vi "Database Configuration Import and Export and Refesh.vi"(8 "error in (no error)":errorcluster, 10 "Database Configuration":T1(ring), 11 "Settings in":refnum<class "Settings.lvclass">) -> (0 "error out":errorcluster, 3 "Settings out":refnum<class "Settings.lvclass">)   [LabVIEW 2023, in "GUI.lvlib" / "Settings.lvlib" / "Settings.lvclass"]
uses:
  Settings.lvclass
  HardwareAbstractionLayer_LVOOP/Database/SQL Public VI/Control/DB Options.ctl
  Settings.lvclass/Settings.ctl
  <vilib>/Utility/file.llb/Read Delimited Spreadsheet (string).vi
  <vilib>/Utility/file.llb/Write Delimited Spreadsheet (string).vi
  HardwareAbstractionLayer_LVOOP/Database/Database.lvclass
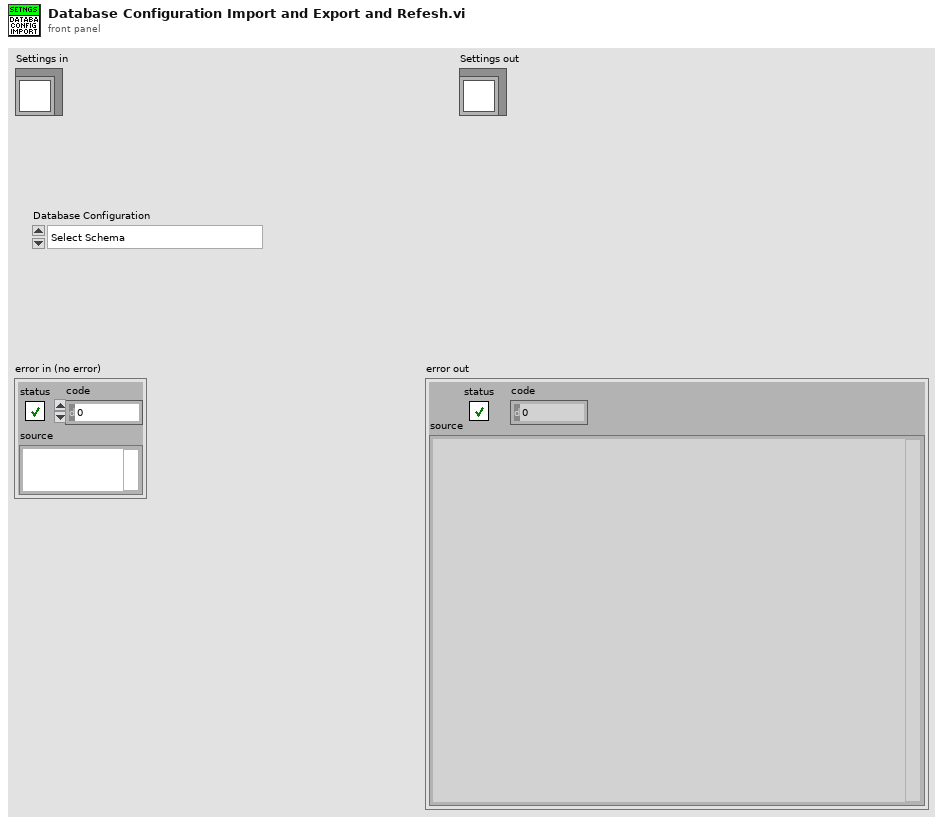
[diagram p1: front panel]
types:
  T1 = enum16{"Select Schema", "Select Table", "Import Table", "Export Table", "Refresh"}
  T2 = typedef "HardwareAbstractionLayer_LVOOP.lvlib/Database.lvclass/DB Options.ctl" = enum16{"Init", "Select Data", "Insert Data", "Update Data", "Delete Data", "Execute Query", "Create Schema", "Create Table", "List Tables", "List Columns", "Close"}
  T3 = cluster{"table":string, "columns":string[], "Data":string[][], "Schema Name":string}
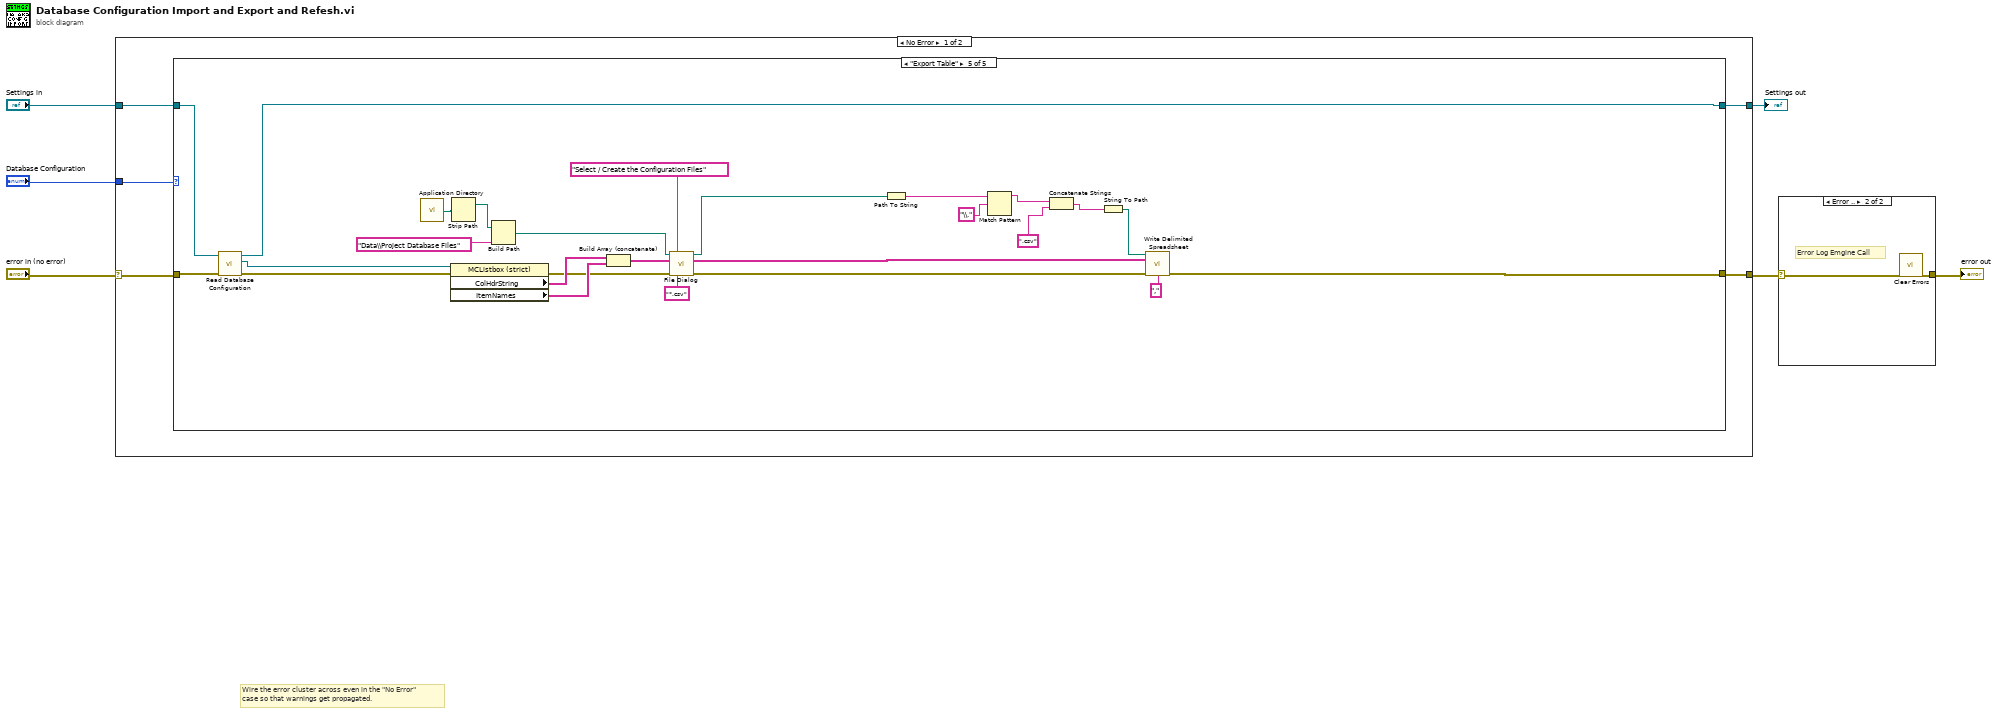
[diagram p0: block diagram]
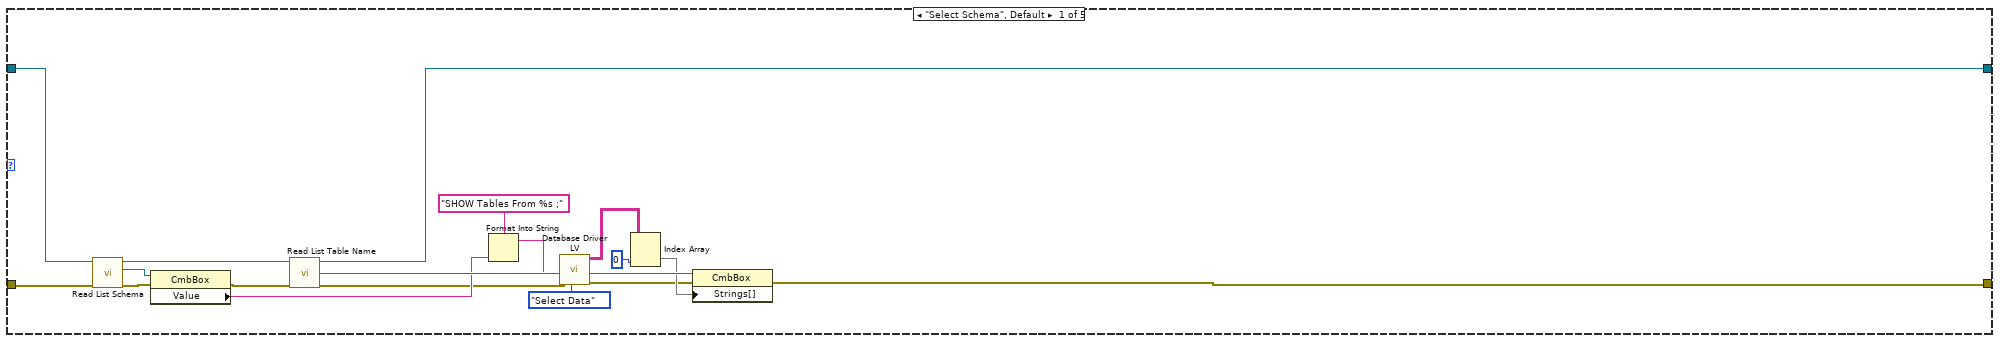
[diagram p3: hidden frame]
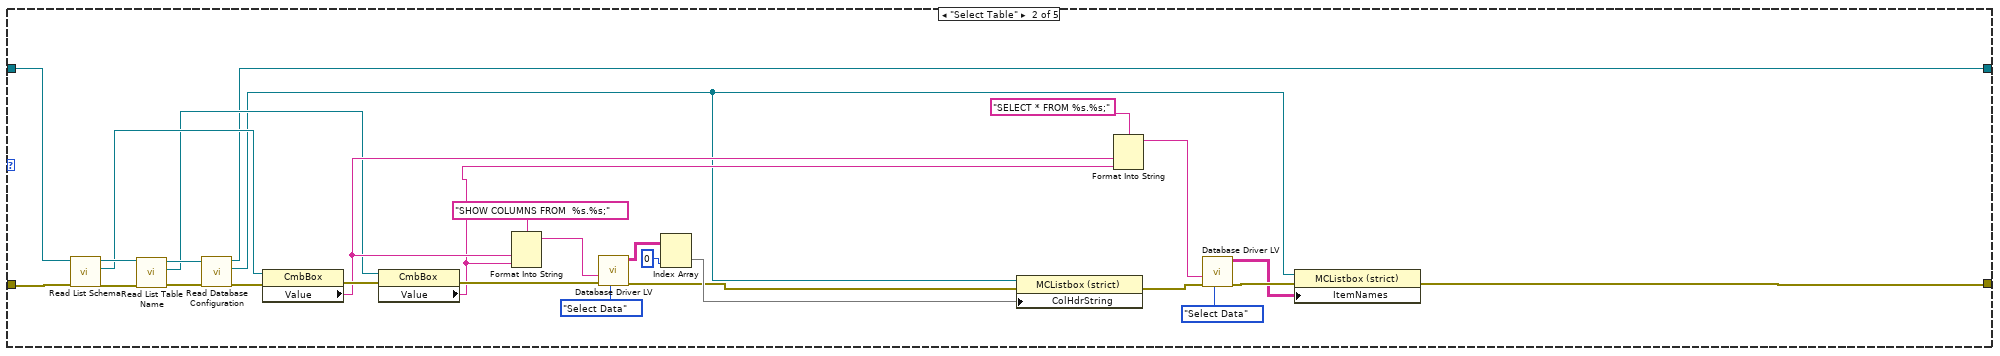
[diagram p4: hidden frame]
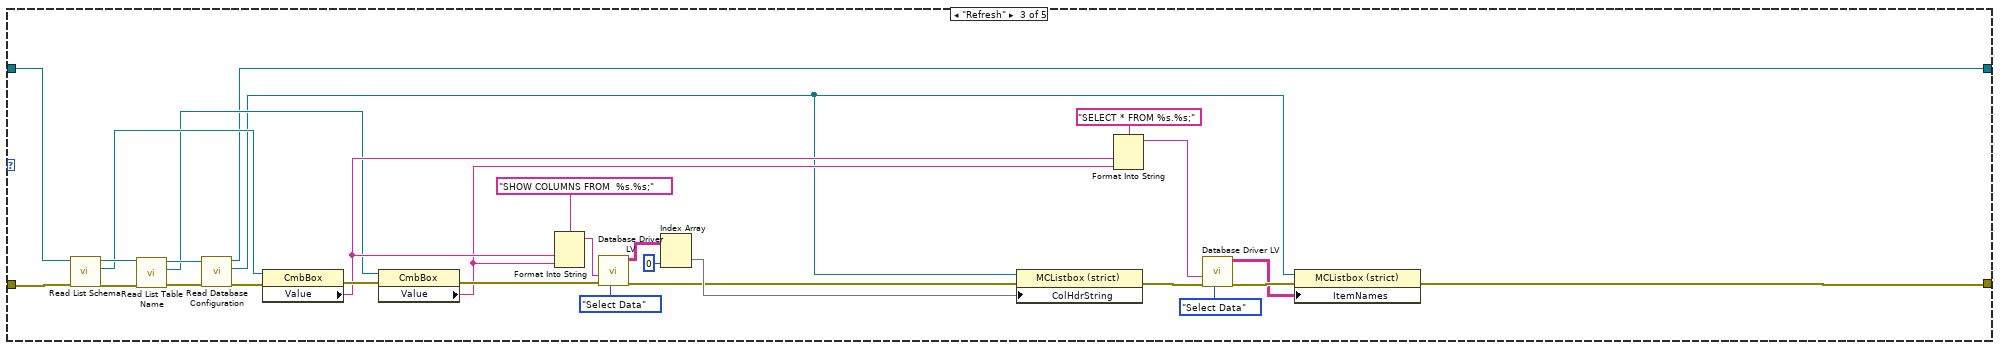
[diagram p5: hidden frame]
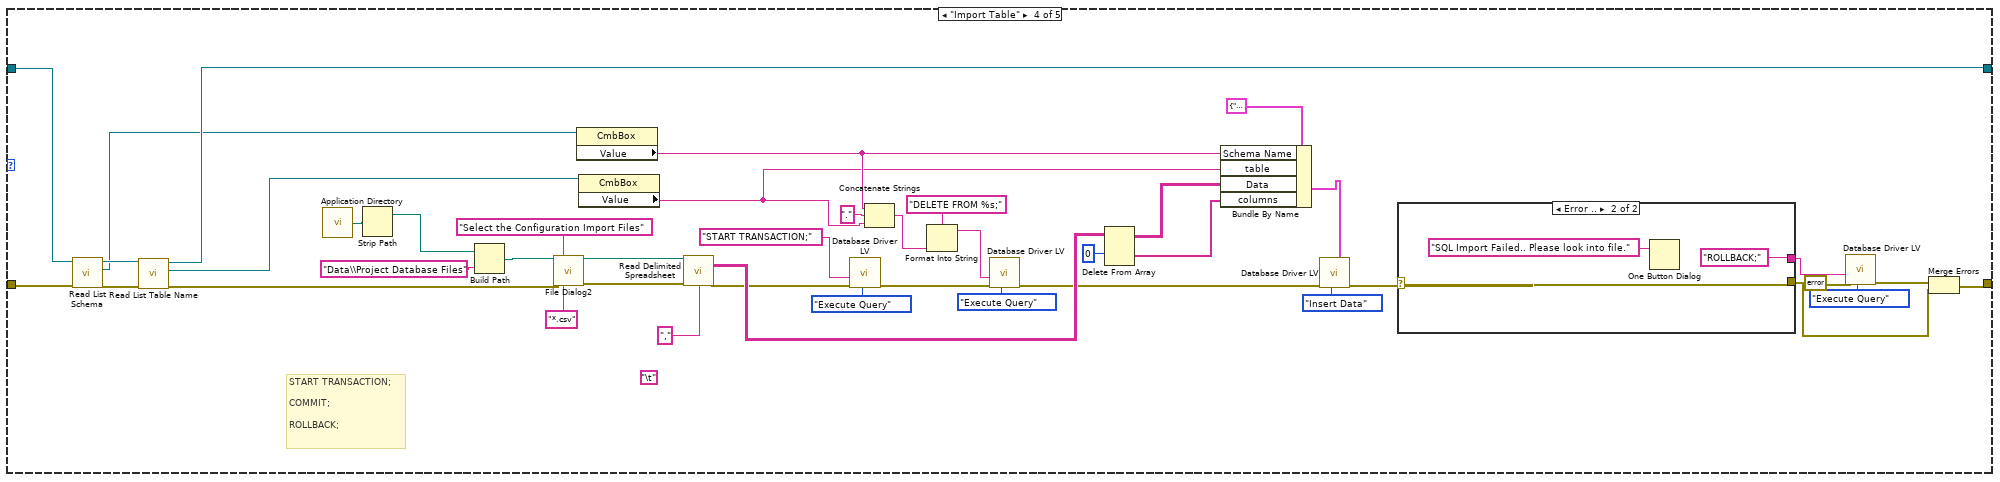
[diagram p6: hidden frame]
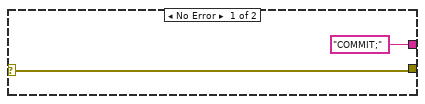
[diagram p7: hidden frame]
diagram:
  # "Wire the error cluster across even in the \"No Error\"\ncase so that warnings get propagated."
  n1 = case shown="No Error" "error in (no error)" {
    selector: "error in (no error)" -> [w8 w162]
    tunnel: [w7 w162] -> w2
    tunnel: [w9 w161] -> w4
    tunnel: "Settings in" -> [w10 w161]
    tunnel: "Database Configuration" -> [w11 _]
    frame No Error {
      n2 = case shown="\"Export Table\"" w11 {
        tunnel: w10 -> [w29 w40 w69 w115 w142]
        tunnel: [w12 w31 w60 w114 w138] -> w9
        tunnel: w8 -> [w28 w41 w70 w116 w141]
        tunnel: [w13 w34 w63 w98 w143] -> w7
        frame "Select Schema", Default {
          n3 = call "Read List Schema.vi"("error in (no error)"=w28, "Settings in"=w29) -> ("error out"=w25:errorcluster, "List Schema"=w26:refnum<vi>, "Settings out"=w27:refnum<class "Settings.lvclass">)  [unwired: 7 in]
          n4 = property class="CmbBox"(reference=w26, error in=w25) -> (error out=w24:errorcluster, "Value"=w17:string)  [unwired: 1 out]
          n5 = call "Read List Table Name.vi"("error in (no error)"=w24, "Settings in"=w27) -> ("error out"=w15:errorcluster, "List Table Name"=w23:refnum<vi>, "Settings out"=w12:refnum<class "Settings.lvclass">)  [unwired: 7 in]
          n6 = Format Into String(format string="SHOW Tables From %s ;" ("SQL query"), w17) -> (resulting string=w20:string)  [unwired: 2 in, 1 out]
          n7 = call "Database Driver LV.vi"("Options"=DB_Options."Select Data", "error in"=w15, "SQL query"=w20) -> ("error out"=w14:errorcluster, "data"=w19:string[][])  [unwired: 5 in, 2 out]
          n8 = Index Array(array=w19, index (col)=0 ("disabled index (col)")) -> (element=w16:string[])  [unwired: 1 in]
          n9 = property class="CmbBox"(reference=w23, error in=w14, "Strings[]"=w16) -> (error out=w13:errorcluster)  [unwired: 1 out]
        }
        frame "Select Table" {
          n10 = call "Read List Schema.vi"("error in (no error)"=w41, "Settings in"=w40) -> ("error out"=w38:errorcluster, "List Schema"=w33:refnum<vi>, "Settings out"=w39:refnum<class "Settings.lvclass">)  [unwired: 7 in]
          n11 = call "Read List Table Name.vi"("error in (no error)"=w38, "Settings in"=w39) -> ("error out"=w37:errorcluster, "List Table Name"=w32:refnum<vi>, "Settings out"=w36:refnum<class "Settings.lvclass">)  [unwired: 7 in]
          n12 = call "Read Database Configuration.vi"("error in (no error)"=w37, "Settings in"=w36) -> ("error out"=w35:errorcluster, "Database Configuration"=w30:refnum<vi>, "Settings out"=w31:refnum<class "Settings.lvclass">)  [unwired: 7 in]
          n13 = property on="Property Node" class="CmbBox"(reference=w33, error in=w35) -> (error out=w53:errorcluster, "Value"=w43:string)  [unwired: 1 out]
          n14 = property on="Property Node" class="CmbBox"(reference=w32, error in=w53) -> (error out=w52:errorcluster, "Value"=w42:string)  [unwired: 1 out]
          n15 = Format Into String(format string="SHOW COLUMNS FROM  %s.%s;" ("SQL query"), w43, w42) -> (resulting string=w58:string)  [unwired: 2 in, 1 out]
          n16 = call "Database Driver LV.vi"("Options"=DB_Options."Select Data", "error in"=w52, "SQL query"=w58) -> ("error out"=w50:errorcluster, "data"=w57:string[][])  [unwired: 5 in, 2 out]
          n17 = Index Array(array=w57, index (col)=0 ("disabled index (col)")) -> (element=w51:string[])  [unwired: 1 in]
          n18 = property on="Property Node" class="MCListbox (strict)"(reference=w30, error in=w50, "ColHdrString"=w51) -> (error out=w48:errorcluster)  [unwired: 1 out]
          n19 = Format Into String(format string="SELECT * FROM %s.%s;", w43, w42) -> (resulting string=w45:string)  [unwired: 2 in, 1 out]
          n20 = call "Database Driver LV.vi"("Options"=DB_Options."Select Data", "error in"=w48, "SQL query"=w45) -> ("error out"=w47:errorcluster, "data"=w44:string[][])  [unwired: 5 in, 2 out]
          n21 = property on="Property Node" class="MCListbox (strict)"(reference=w30, error in=w47, "ItemNames"=w44) -> (error out=w34:errorcluster)  [unwired: 1 out]
        }
        frame "Refresh" {
          n22 = call "Read List Schema.vi"("error in (no error)"=w70, "Settings in"=w69) -> ("error out"=w67:errorcluster, "List Schema"=w62:refnum<vi>, "Settings out"=w68:refnum<class "Settings.lvclass">)  [unwired: 7 in]
          n23 = call "Read List Table Name.vi"("error in (no error)"=w67, "Settings in"=w68) -> ("error out"=w66:errorcluster, "List Table Name"=w61:refnum<vi>, "Settings out"=w65:refnum<class "Settings.lvclass">)  [unwired: 7 in]
          n24 = call "Read Database Configuration.vi"("error in (no error)"=w66, "Settings in"=w65) -> ("error out"=w64:errorcluster, "Database Configuration"=w59:refnum<vi>, "Settings out"=w60:refnum<class "Settings.lvclass">)  [unwired: 7 in]
          n25 = property on="Property Node" class="CmbBox"(reference=w62, error in=w64) -> (error out=w82:errorcluster, "Value"=w72:string)  [unwired: 1 out]
          n26 = property on="Property Node" class="CmbBox"(reference=w61, error in=w82) -> (error out=w81:errorcluster, "Value"=w71:string)  [unwired: 1 out]
          n27 = Format Into String(format string="SHOW COLUMNS FROM  %s.%s;" ("SQL query"), w72, w71) -> (resulting string=w87:string)  [unwired: 2 in, 1 out]
          n28 = call "Database Driver LV.vi"("Options"=DB_Options."Select Data", "error in"=w81, "SQL query"=w87) -> ("error out"=w79:errorcluster, "data"=w86:string[][])  [unwired: 5 in, 2 out]
          n29 = Index Array(array=w86, index (col)=0 ("disabled index (col)")) -> (element=w80:string[])  [unwired: 1 in]
          n30 = property on="Property Node" class="MCListbox (strict)"(reference=w59, error in=w79, "ColHdrString"=w80) -> (error out=w77:errorcluster)  [unwired: 1 out]
          n31 = Format Into String(format string="SELECT * FROM %s.%s;", w72, w71) -> (resulting string=w74:string)  [unwired: 2 in, 1 out]
          n32 = call "Database Driver LV.vi"("Options"=DB_Options."Select Data", "error in"=w77, "SQL query"=w74) -> ("error out"=w76:errorcluster, "data"=w73:string[][])  [unwired: 5 in, 2 out]
          n33 = property on="Property Node" class="MCListbox (strict)"(reference=w59, error in=w76, "ItemNames"=w73) -> (error out=w63:errorcluster)  [unwired: 1 out]
        }
        frame "Import Table" {
          (unwired) "\t"
          # "START TRANSACTION;\n\nCOMMIT;\n\nROLLBACK;"
          n34 = call "Read List Schema.vi"("error in (no error)"=w116, "Settings in"=w115) -> ("error out"=w117:errorcluster, "List Schema"=w113:refnum<vi>, "Settings out"=w118:refnum<class "Settings.lvclass">)  [unwired: 7 in]
          n35 = call "Read List Table Name.vi"("error in (no error)"=w117, "Settings in"=w118) -> ("error out"=w88:errorcluster, "List Table Name"=w112:refnum<vi>, "Settings out"=w114:refnum<class "Settings.lvclass">)  [unwired: 7 in]
          n36 = call <vilib>:"Application Directory.vi"() -> ("Application Directory"=w122:path)
          n37 = Strip Path(path=w122) -> (stripped path=w121:path)  [unwired: 1 out]
          n38 = Build Path(base path=w121, name or relative path="Data\\Project Database Files") -> (appended path=w119:path)
          n39 = call "File Dialog2"("start path"=w119, "prompt"="Select the Configuration Import Files", "error in"=w88, "pattern (all files)"="*.csv" ("pattern label")) -> ("selected path"=w125:path, "error out"=w126:errorcluster)  [unwired: 8 in, 2 out]
          n40 = property on="Property Node" class="CmbBox"(reference=w113) -> ("Value"=w90:string)  [unwired: 1 in, 2 out]
          n41 = property on="Property Node" class="CmbBox"(reference=w112) -> ("Value"=w89:string)  [unwired: 1 in, 2 out]
          n42 = call-poly <vilib>:"Read Delimited Spreadsheet.vi"("file path (dialog if empty)"=w125, "error in (no error)"=w126, "delimiter (\\t)"="," ("delimiter (\\t)")) -> ("all rows"=w129:string[][], "error out"=w104:errorcluster)  [unwired: 7 in, 4 out]
          n43 = call "Database Driver LV.vi"("Options"=DB_Options."Execute Query", "error in"=w104, "SQL query"="START TRANSACTION;") -> ("error out"=w103:errorcluster)  [unwired: 5 in, 3 out]
          n44 = Concatenate Strings(w90, "." ("element"), w89) -> (w108:string)
          n45 = Format Into String(format string="DELETE FROM %s;" ("SQL query"), w108) -> (resulting string=w107:string)  [unwired: 2 in, 1 out]
          n46 = call "Database Driver LV.vi"("Options"=DB_Options."Execute Query", "error in"=w103, "SQL query"=w107) -> ("error out"=w111:errorcluster)  [unwired: 5 in, 3 out]
          n47 = Delete From Array(array=w129, index (row)=0) -> (deleted portion=w128:string[], array with subset deleted=w93:string[][])  [unwired: 2 in]
          n48 = Bundle By Name(cluster=T3 {"table"="", "columns"=[], "Data"=[], "Schema Name"=""} ("Insert Data"), "Schema Name"=w90, "table"=w89, "Data"=w93, "columns"=w128) -> (w91:T3)
          n49 = call "Database Driver LV.vi"("Insert Data"=w91, "Options"=DB_Options."Insert Data", "error in"=w111) -> ("error out"=w101:errorcluster)  [unwired: 5 in, 3 out]
          n50 = case shown="Error .." w101 {
            selector: w101 -> [w132 w134]
            tunnel: [w132 w134] -> w97
            tunnel: ["COMMIT;" "ROLLBACK;"] -> w96
            frame No Error {
            }
            frame Error {
              n51 = One Button Dialog(message="SQL Import Failed.. Please look into file.") -> ()  [unwired: 1 in, 1 out]
            }
          }
          n52 = call "Database Driver LV.vi"("Options"=DB_Options."Execute Query", "error in"=errorcluster {"status"=FALSE, "code"=0, "source"=""}, "SQL query"=w96) -> ("error out"=w99:errorcluster)  [unwired: 5 in, 3 out]
          n53 = Merge Errors(w99, w97) -> (w98:errorcluster)
        }
        frame "Export Table" {
          n54 = call "Read Database Configuration.vi"("error in (no error)"=w141, "Settings in"=w142) -> ("error out"=w140:errorcluster, "Database Configuration"=w139:refnum<vi>, "Settings out"=w138:refnum<class "Settings.lvclass">)  [unwired: 7 in]
          n55 = call <vilib>:"Application Directory.vi"() -> ("Application Directory"=w155:path)
          n56 = property on="Property Node" class="MCListbox (strict)"(reference=w139, error in=w140) -> (error out=w157:errorcluster, "ColHdrString"=w159:string[], "ItemNames"=w160:string[][])  [unwired: 1 out]
          n57 = Strip Path(path=w155) -> (stripped path=w154:path)  [unwired: 1 out]
          n58 = Build Path(base path=w154, name or relative path="Data\\Project Database Files") -> (appended path=w153:path)
          n59 = Build Array (concatenate)(w159, w160) -> (w158:string[][])
          n60 = call "File Dialog"("start path"=w153, "prompt"="Select / Create the Configuration Files", "error in"=w157, "pattern (all files)"="*.csv") -> ("selected path"=w152:path, "error out"=w156:errorcluster)  [unwired: 8 in, 2 out]
          n61 = Path To String(path=w152) -> (string=w151:string)
          n62 = Match Pattern(string=w151, regular expression="\\." ("pattern (all files)")) -> (before substring=w150:string)  [unwired: 1 in, 3 out]
          n63 = Concatenate Strings(w150, ".csv" ("string")) -> (w149:string)
          n64 = String To Path(string=w149) -> (path=w148:path)
          n65 = call-poly <vilib>:"Write Delimited Spreadsheet.vi"("file path (dialog if empty)"=w148, "2D data"=w158, "error in (no error)"=w156, "delimiter (\\t)"="," ("delimiter (\\t)")) -> ("error out"=w143:errorcluster)  [unwired: 10 in, 1 out]
        }
      }
    }
    frame Error {
    }
  }
  "Settings out" <- w4
  n66 = case shown="Error .." w2 {
    selector: w2 -> [w163 w165]
    tunnel: [w163 w164] -> w1
    frame No Error {
    }
    frame Error {
      # "Error Log Emgine Call"
      n67 = call <vilib>:"Clear Errors.vi"("error in (no error)"=w165) -> ("error out"=w164:errorcluster)  [unwired: 5 in, 1 out]
    }
  }
  "error out" <- w1
